vi "Motors Close.vi"(2 "error in":errorcluster, 3 "VISA in":refnum<visa-resource-name>="COM7") -> (0 "error out":errorcluster)   [LabVIEW 2018]
panel:
  in  "Eanble 4":bool
  in  "Enable 3":bool
  in  "Enable 2":bool
  in  "Enable 1":bool
  out "read buffer 4":string
  out "read buffer 3":string
  out "read buffer 2":string
  out "read buffer 1":string
  in  "Closing command 4":string="4ID"
  in  "Closing command 3":string="3ID"
  in  "Closing command 2":string="2ID"
  in  "Closing command 1":string="1ID"
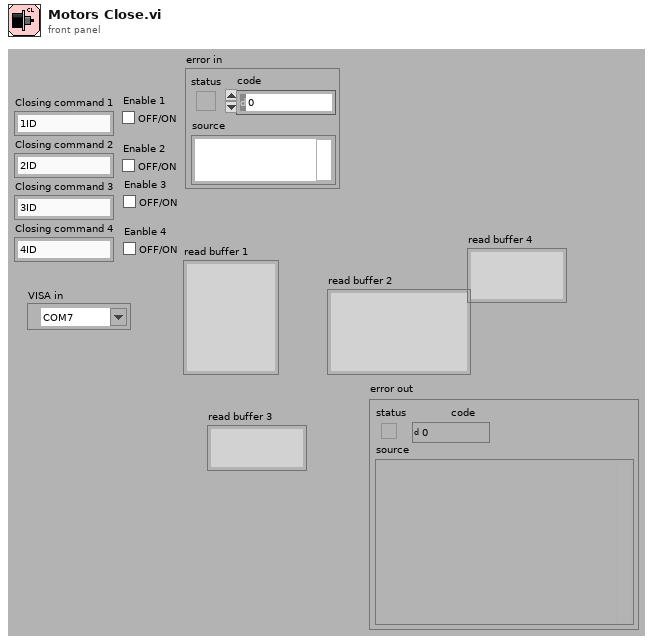
[diagram p1: front panel]
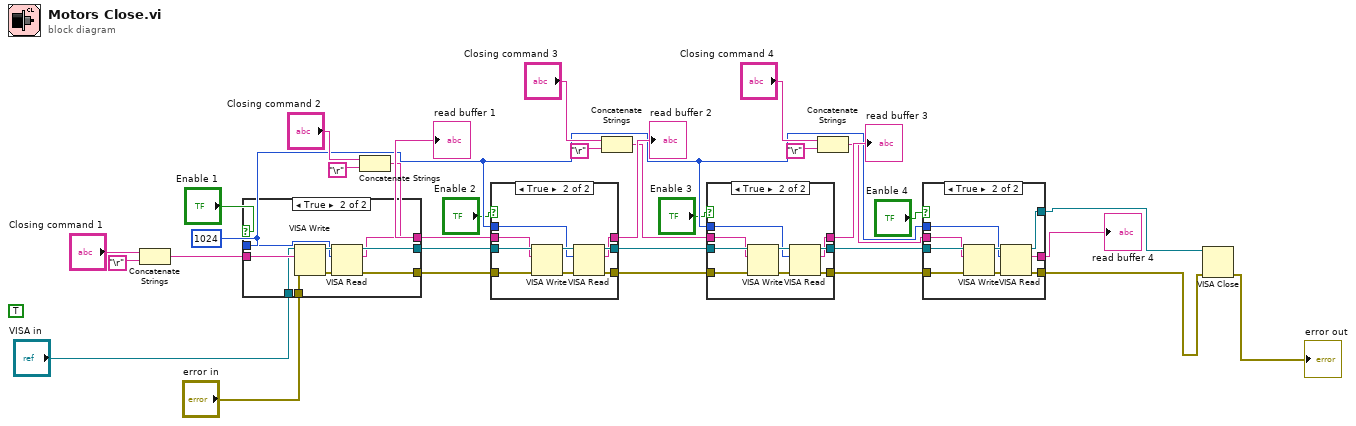
[diagram p0: block diagram]
diagram:
  w10 = u32 1024 ("byte count")
  (unwired) TRUE
  n1 = Concatenate Strings("Closing command 1", "\r") -> (w21:string)
  n2 = case shown="True" "Enable 1" {
    tunnel: [w33 w41] -> w24
    tunnel: [w34 w40] -> w23
    tunnel: w10 -> [_ w39]
    tunnel: [_ w38] -> w22
    tunnel: w21 -> [_ w37]
    tunnel: "VISA in" -> [w33 w36]
    tunnel: "error in" -> [w34 w35]
    frame False {
    }
    frame True {
      n3 = VISA Write(VISA resource name=w36, write buffer=w37, error in (no error)=w35) -> (VISA resource name out=w42:refnum<visa-resource-name>, error out=w43:errorcluster)  [unwired: 1 out]
      n4 = VISA Read(VISA resource name=w42, byte count=w39, error in (no error)=w43) -> (VISA resource name out=w41:refnum<visa-resource-name>, read buffer=w38:string, error out=w40:errorcluster)  [unwired: 1 out]
    }
  }
  "read buffer 1" <- w22
  n5 = Concatenate Strings("Closing command 2", "\r") -> (w19:string)
  n6 = case shown="True" "Enable 2" {
    tunnel: w24 -> [w45 w53]
    tunnel: w23 -> [w44 w50]
    tunnel: [w45 w51] -> w18
    tunnel: [w44 w49] -> w17
    tunnel: w10 -> [_ w48]
    tunnel: [_ w47] -> w20
    tunnel: w19 -> [_ w46]
    frame False {
    }
    frame True {
      n7 = VISA Write(VISA resource name=w53, write buffer=w46, error in (no error)=w50) -> (VISA resource name out=w52:refnum<visa-resource-name>, error out=w54:errorcluster)  [unwired: 1 out]
      n8 = VISA Read(VISA resource name=w52, byte count=w48, error in (no error)=w54) -> (VISA resource name out=w51:refnum<visa-resource-name>, read buffer=w47:string, error out=w49:errorcluster)  [unwired: 1 out]
    }
  }
  "read buffer 2" <- w20
  n9 = Concatenate Strings("Closing command 3", "\r") -> (w15:string)
  n10 = case shown="True" "Enable 3" {
    tunnel: w18 -> [w56 w64]
    tunnel: [w56 w62] -> w14
    tunnel: w17 -> [w55 w61]
    tunnel: [w55 w60] -> w13
    tunnel: w10 -> [_ w59]
    tunnel: [_ w58] -> w16
    tunnel: w15 -> [_ w57]
    frame False {
    }
    frame True {
      n11 = VISA Write(VISA resource name=w64, write buffer=w57, error in (no error)=w61) -> (VISA resource name out=w63:refnum<visa-resource-name>, error out=w65:errorcluster)  [unwired: 1 out]
      n12 = VISA Read(VISA resource name=w63, byte count=w59, error in (no error)=w65) -> (VISA resource name out=w62:refnum<visa-resource-name>, read buffer=w58:string, error out=w60:errorcluster)  [unwired: 1 out]
    }
  }
  "read buffer 3" <- w16
  n13 = Concatenate Strings("Closing command 4", "\r") -> (w11:string)
  n14 = case shown="True" "Eanble 4" {
    tunnel: w14 -> [w67 w75]
    tunnel: w13 -> [w66 w73]
    tunnel: [w67 w72] -> w1
    tunnel: [w66 w71] -> w3
    tunnel: [_ w70] -> w12
    tunnel: w11 -> [_ w69]
    tunnel: w10 -> [_ w68]
    frame False {
    }
    frame True {
      n15 = VISA Write(VISA resource name=w75, write buffer=w69, error in (no error)=w73) -> (VISA resource name out=w74:refnum<visa-resource-name>, error out=w76:errorcluster)  [unwired: 1 out]
      n16 = VISA Read(VISA resource name=w74, byte count=w68, error in (no error)=w76) -> (VISA resource name out=w72:refnum<visa-resource-name>, read buffer=w70:string, error out=w71:errorcluster)  [unwired: 1 out]
    }
  }
  "read buffer 4" <- w12
  n17 = VISA Close(VISA resource name=w1, error in (no error)=w3) -> (error out=→"error out":errorcluster)
